vi "Get VI Static Refnum.vi"(8 "error in (no error)":errorcluster, 11 "Console Reply in":refnum<class "Console Reply.lvclass">) -> (0 "error out":errorcluster, 2 "VI Static Refnum":refnum<vi>, 3 "Console Reply out":refnum<class "Console Reply.lvclass">)   [LabVIEW 2015, in "EditPanel API.lvlib" / "Console Reply.lvclass"]
uses:
  Console Reply.lvclass
  Console Reply.lvclass/Console Reply.ctl
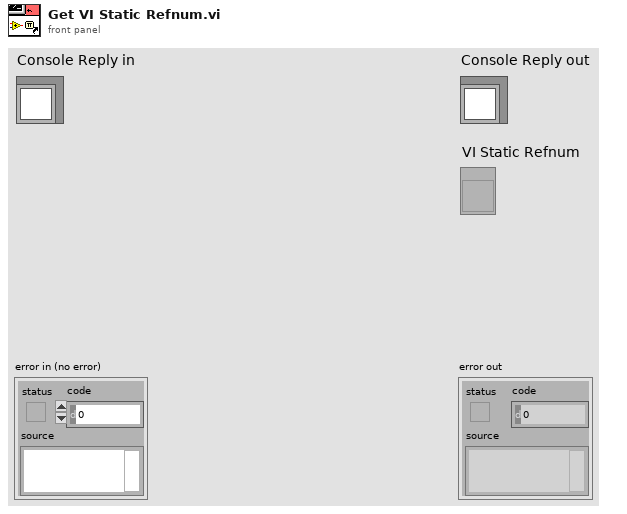
[diagram p1: front panel]
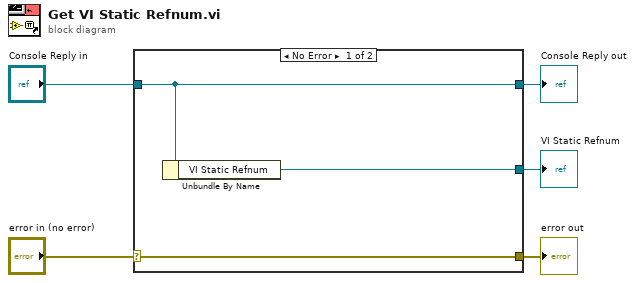
[diagram p0: block diagram]
diagram:
  n1 = case shown="No Error" "error in (no error)" {
    selector: "error in (no error)" -> [w8 w9]
    tunnel: [w8 w9] -> w4
    tunnel: [w7 w10] -> w2
    tunnel: "Console Reply in" -> [w7 w10]
    tunnel: [w6 _] -> w1
    frame No Error {
      n2 = Unbundle By Name(w7) -> ("VI Static Refnum"=w6:refnum<vi>)
    }
    frame Error {
    }
  }
  "error out" <- w4
  "Console Reply out" <- w2
  "VI Static Refnum" <- w1
